vi "Oscilloscope.vi"() -> ()   [LabVIEW 2025]
uses:
  <vilib>/Instr/_visa.llb/VISA Configure Serial Port (Instr).vi
panel:
  in  "?":bool
  in  "Tab Control":enum32{"Page 1"}(tab)
  in  "VISA resource name":refnum<visa-resource-name>
  in  "Volt/Div":dbl(knob) scale=0.1..10.0
  in  "Time/Div":dbl(knob) scale=0.1..10.0
  in  "Trigger mode":enum16{"Auto", "Normal", "Single"}(ring)
  in  "Trigger level":dbl
  out "Waveform Chart":dbl(graph)
  in  "?":bool
  in  "?":dbl
  in  "Numeric 2":dbl
  out "Boolean":bool
  in  "Multiplier":dbl
  out "String":string
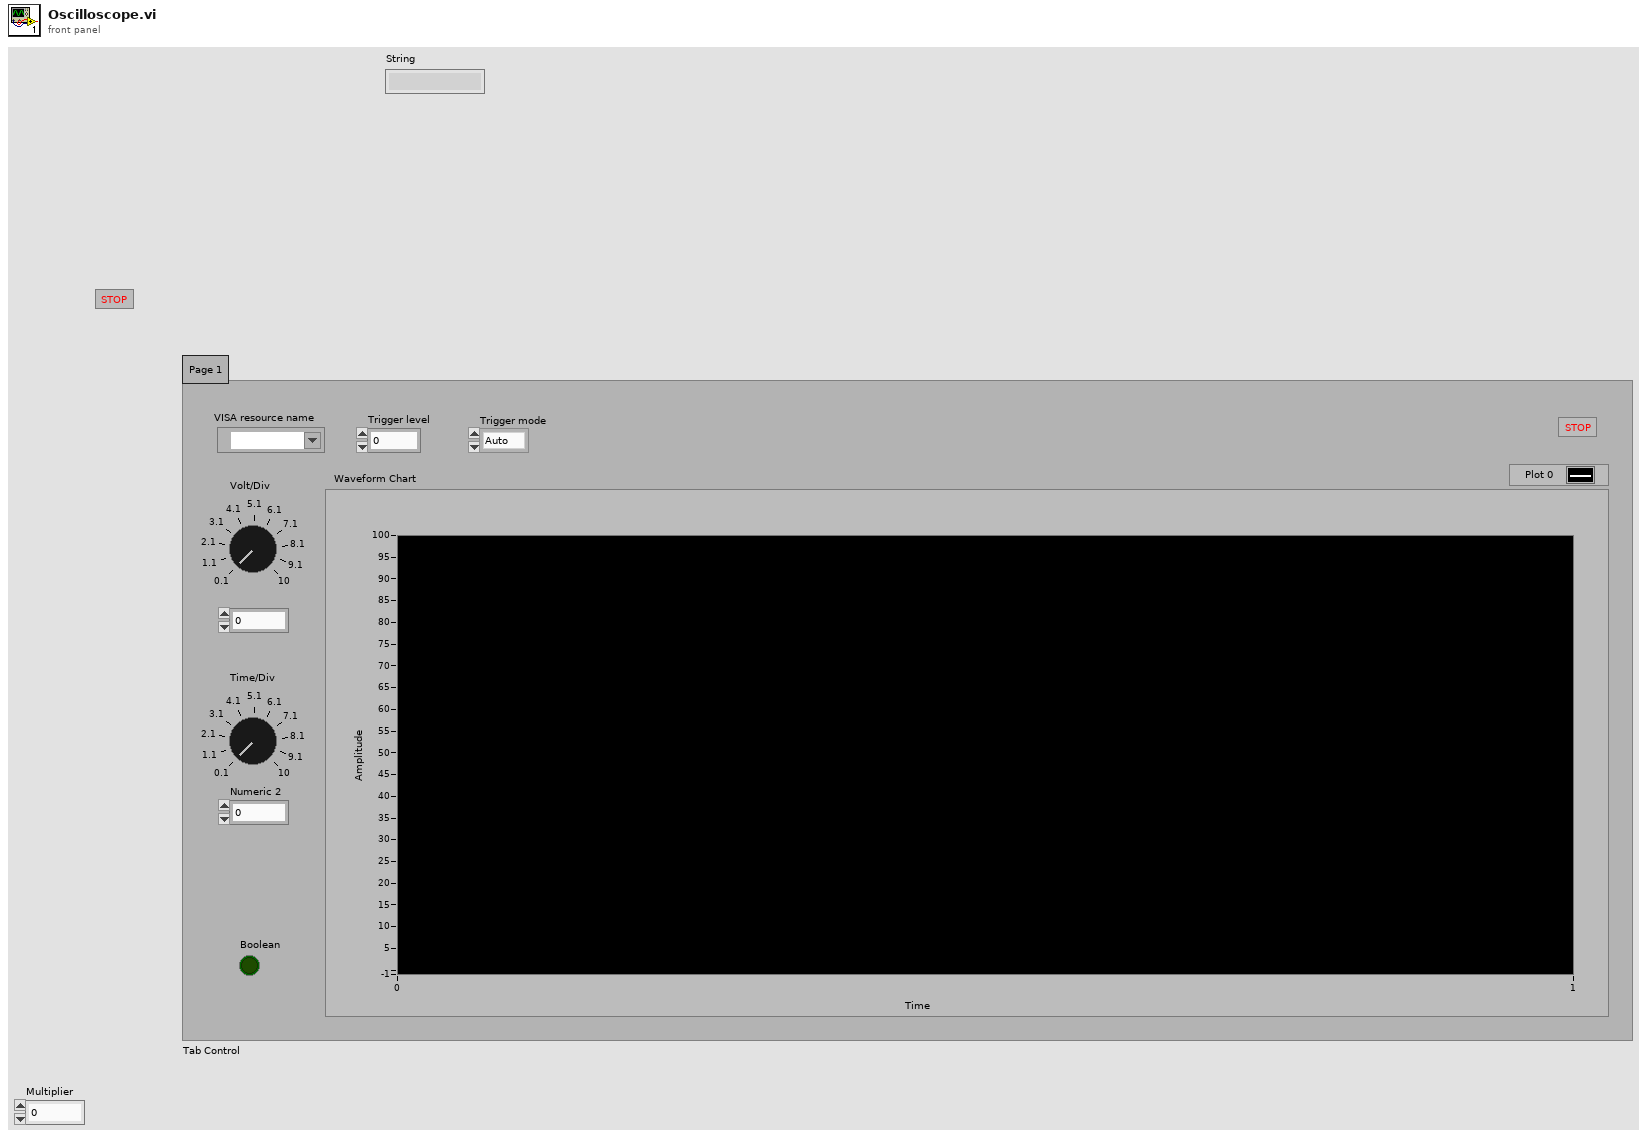
[diagram p1: front panel]
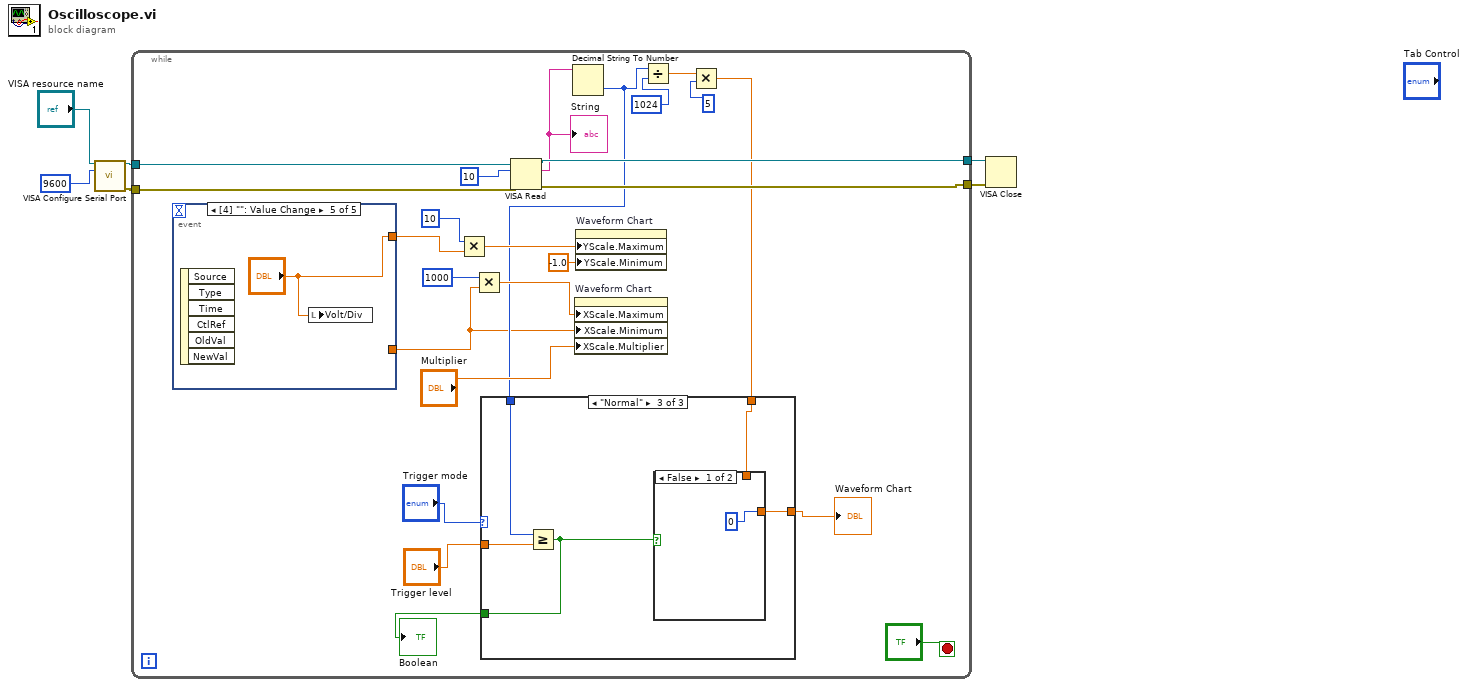
[diagram p0: block diagram]
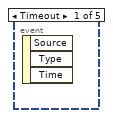
[diagram p2: hidden frame]
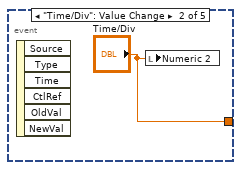
[diagram p3: hidden frame]
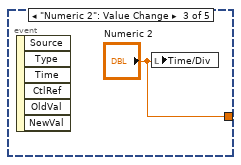
[diagram p4: hidden frame]
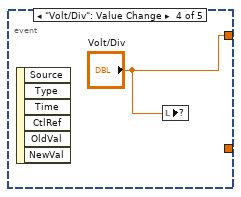
[diagram p5: hidden frame]
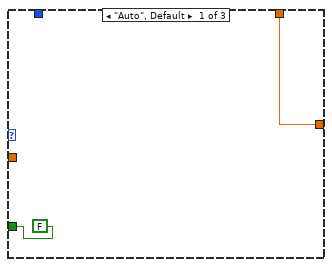
[diagram p6: hidden frame]
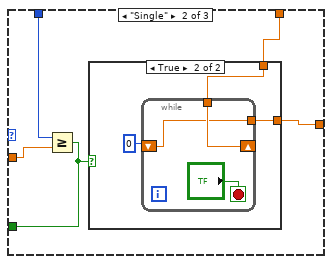
[diagram p7: hidden frame]
diagram:
  n1 = call-poly "VISA Configure Serial Port"("VISA resource name"="VISA resource name", "baud rate (9600)"=9600) -> ("VISA resource name out"=w5:refnum<visa-resource-name>, "error out"=w4:errorcluster)  [unwired: 12 in]
  n2 = while {
    tunnel: w5 -> [w29]
    tunnel: w4 -> [w28]
    tunnel: [w27] -> w3
    tunnel: [w26] -> w2
    stop <- "?" stop-if-true
    n3 = event shown="[4] \"\": Value Change" {
      selector: _ -> [_ _ _ _ _]
      dyn-events: _ -> [_ _ _ _ _]
      timeout: _ -> [_ _ _ _ _]
      tunnel: [_ _ _ "Volt/Div" "?"] -> w10
      tunnel: [_ "Time/Div" "Numeric 2" _ _] -> w9
      event Timeout {
        n4 = event-data() -> ()  [unwired: 1 in, 3 out]
      }
      event "Time/Div": Value Change {
        n5 = event-data() -> ()  [unwired: 1 in, 6 out]
        n6 = local write "Numeric 2"("Time/Div") -> ()
      }
      event "Numeric 2": Value Change {
        n7 = event-data() -> ()  [unwired: 1 in, 6 out]
        n8 = local write "Time/Div"("Numeric 2") -> ()
      }
      event "Volt/Div": Value Change {
        n9 = event-data() -> ()  [unwired: 1 in, 6 out]
        n10 = local write item#11("Volt/Div") -> ()
      }
      event Value Change {
        n11 = event-data() -> ()  [unwired: 1 in, 6 out]
        n12 = local write "Volt/Div"("?") -> ()
      }
    }
    n13 = Multiply(x=10, y=w10) -> (x*y=w19:dbl)
    n14 = Multiply(x=1000, y=w9) -> (x*y=w17:dbl)
    n15 = VISA Read(VISA resource name=w29, byte count=10, error in (no error)=w28) -> (VISA resource name out=w27:refnum<visa-resource-name>, read buffer=w22:string, error out=w26:errorcluster)  [unwired: 1 out]
    "String" <- w22
    n16 = Decimal String To Number(string=w22) -> (number=w13:i32)  [unwired: 2 in, 1 out]
    n17 = property on="Waveform Chart" class="WFChart (strict)"("XScale.Maximum"=w17, "XScale.Minimum"=w9, "XScale.Multiplier"="Multiplier") -> ()  [unwired: 2 in, 2 out]
    n18 = property on="Waveform Chart" class="WFChart (strict)"("YScale.Maximum"=w19, "YScale.Minimum"=-1.0 ("Y Scale.Range:Minimum")) -> ()  [unwired: 2 in, 2 out]
    n19 = Divide(x=w13, y=1024) -> (x/y=w25:dbl)
    n20 = Multiply(x=w25, y=5) -> (x*y=w8:dbl)
    n21 = case shown="\"Normal\"" "Trigger mode" {
      tunnel: w8 -> [w36 w40 w51]
      tunnel: [w36 w39 w50] -> w14
      tunnel: w13 -> [_ w41 w53]
      tunnel: "Trigger level" -> [_ w38 w52]
      tunnel: [FALSE w37 w49] -> w7
      frame "Auto", Default {
      }
      frame "Single" {
        n22 = Greater Or Equal?(x=w41, y=w38) -> (x >= y?=w37:bool)
        n23 = case shown="True" w37 {
          tunnel: w40 -> [w42 w45]
          tunnel: [w42 w43] -> w39
          frame False {
          }
          frame True {
            n24 = while {
              shift-right: [w47] -> _
              shift-left: 0 -> [w46]
              tunnel: w45 -> [w47]
              tunnel: [w46] -> w43
              stop <- "?" stop-if-true
            }
          }
        }
      }
      frame "Normal" {
        n25 = Greater Or Equal?(x=w53, y=w52) -> (x >= y?=w49:bool)
        n26 = case shown="False" w49 {
          tunnel: w51 -> [_ w55]
          tunnel: [0 w55] -> w50
          frame False {
          }
          frame True {
          }
        }
      }
    }
    "Waveform Chart" <- w14
    "Boolean" <- w7
  }
  n27 = VISA Close(VISA resource name=w3, error in (no error)=w2) -> ()  [unwired: 1 out]
